vi "Pack Launch Nested Models Msg.vi"(10 "Models":refnum<class "IModel.lvclass">[](array[class])) -> (3 "Launch Nested Models Msg":refnum<class "Launch Nested Models Msg.lvclass">)   [LabVIEW 2017, in "IModel.lvlib" / "Launch Nested Models Msg.lvclass"]
uses:
  Launch Nested Models Msg.lvclass
  IModel/IModel.lvclass
  C:/Program Files (x86)/National Instruments/LabVIEW 2017/vi.lib/ActorFramework/Actor/Actor.lvclass
  Launch Nested Models Msg.lvclass/Launch Nested Models Msg.ctl
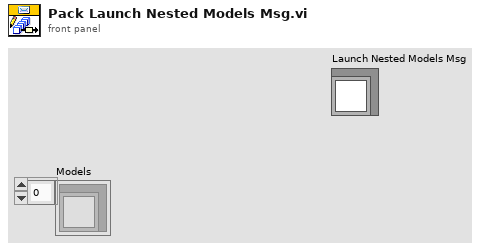
[diagram p1: front panel]
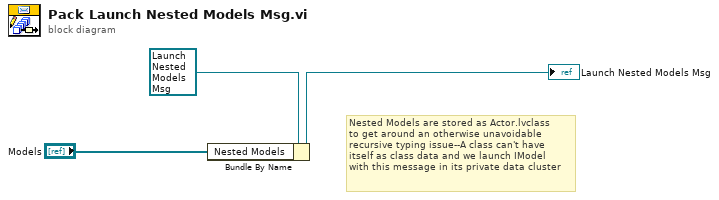
[diagram p0: block diagram]
diagram:
  # "Nested Models are stored as Actor.lvclass\nto get around an otherwise unavoidable\nrecursive typing issue--A class can't have\nitself as class data and we launch IModel\nwith this message in its private data cluster"
  n1 = Bundle By Name(cluster=refnum<class "Launch Nested Models Msg.lvclass"> refnum ("Launch Nested Models Msg"), "Nested Models"="Models") -> (→"Launch Nested Models Msg":refnum<class "Launch Nested Models Msg.lvclass">)
